vi "winchcontrol2014_preT-Tide_Altimeter_withTime.vi"() -> ()   [LabVIEW 2014]
uses:
  Instance           1 20Saved   winchcontrol .vi
  Instance           2 20Saved   winchcontrol .vi
  Instance           4 20Saved   winchcontrol .vi
  Instance           3 20Saved   winchcontrol .vi
  Instance           5 20Saved   winchcontrol .vi
  Instance           6 20Saved   winchcontrol .vi
panel:
  in  "pressure num":dbl
  out "Dz/Dt":T1(graph)
  in  "VelOut Fact.[turns/s]":dbl=4.2 min=0.0 max=8.0 step=0.1 format="%_2f"
  out "Depth History":T2(graph)
  out "Conductivity":T1(graph)
  out "Alti Range":T1(graph)
  in  "Path of Image Capture":path=path "/OPG_Winch_MiniCoreDuo/Users/opg/Sites/FCTD_WINCH/LabView.png"
  in  "Screen Capture":bool
  out "Last update string":string="Updated: 10/29/12 6:37:41 PM"
  in  "Port":i32=4050
  in  "Red Lion IP Address":string="192.168.1.160"
  in  "Beep\non wait?":bool=TRUE
  in  "Drive by \nCTD Data":bool=TRUE
  out "isMaxPaySet":bool
  out "Old Max Payout":dbl=500.0
  in  "Max. depth [m]":dbl=330.0 min=0.0 max=2000.0 step=1.0 format="%#_4f"
  out "Time @ max":timestamp=timestamp(3434357554.995505 s since 1904-01-01) format="%<%H:%M:%S>T"
  out "Max payout":dbl=26.1 format="%#_6f"
  out "Max depth":dbl format="%#_6f"
  in  "Go Up Now":bool
  in  "Final In Speed\n[turns/sec]":dbl=0.7 min=0.0 max=4.0 step=0.1 format="%_2f"
  in  "Slow depth\n[turns]":dbl=7.0 min=0.0 max=1500.0 step=1.0
  out "Final in Speed":dbl=0.7 min=0.0 max=4.0 step=0.1 format="%3_2g"
  out "Slow Depth":dbl=7.0 min=0.0 max=4.0 step=0.1
  out "CTD Com Miss Count":dbl
  out "Winch Com Miss Count":dbl=1.0
  out "Sax Status":u8[](array[numeric])=[1, 1, 0, 0, 5, 0, 1, 1, 0, 0]
  out "Pressure":T1(graph)
  out "i value":i32
  out "concatenated string":string="$OPGST,1,2,1243"
  out "CTD data":string="2615984408,1.818078,23.842880,5.097004"
  out "Depth":dbl(slide)=1.8080824462346528 min=0.0 max=1200.0 scale format="%#_4f"
  out "*(type *) &x":i32=38
  out "timestamp":u32=2615984408
  out "Temperature":T1(graph)
  out "Parameter String":string="$reqparmx:0019;0000$OPGWPM,10,16,+   6,+ 500, 4.2, 2.0,10000,10000,20000,40000,60000,60000,    0.70,    7,;"
  out "Status String":string="$OPGWST,3,1,+   1.8, 266.9,   0,- 0.01,   0.00,   0,   26307,;"
  out "Sax Status Code":dbl=26307.0 format="%#_8f"
  out "Motor Current":dbl
  out "Motor Payout":dbl=266.9
  out "Sheave Payout":dbl
  out "ATM90 Payout":dbl=1.8
  in  "CTD Data  IP Address":string="192.168.1.158"
  in  "Port":i32=2342
  out "bytes written":i32=62
  out "RL Status Received":bool=TRUE
  out "Acc Out":dbl=10000.0
  out "Acc In":dbl=10000.0
  out "Winch Action Status":T3(ring)=enum."HOMING"
  out "Winch Control Mode":u16(ring)=3 items=["STOPPED", "MANUAL JOY", "MANUAL POT", "AUTO", "SEMIAUTO"]
  out "Decel Stop In":dbl=60000.0
  out "Decel Stop Out":dbl=60000.0
  out "Decel In":dbl=40000.0
  out "Decel Out":dbl=20000.0
  out "Wire In Speed":dbl=2.0
  out "Wire Out Speed":dbl=4.2
  out "Min Payout":dbl=6.0
  out "Max Payout":dbl=500.0
  out "I Limit Out":dbl=10.0
  out "I Limit In":dbl=16.0
  in  "Drop time [min.]":dbl=8.099999999999985 min=0.0 step=0.1 format="%.1f"
  out "output":string
  in  "Stop Now":bool
  in  "Wire In Speed\n[turns/sec]":dbl=2.0 min=0.0 max=5.0 step=0.1 format="%3_2f"
  in  "Decel in":dbl=40000.0
  in  "Decel out":dbl=20000.0
  in  "Stop decel in":dbl=60000.0
  in  "Stop decel out":dbl=60000.0
  in  "Accel  in":dbl=10000.0
  in  "Accel out":dbl=10000.0
  in  "Current limit out\n[Amps]":dbl=10.0 min=0.0 max=20.0 step=0.1 format="%_3f"
  in  "Current limit in\n[Amps]":dbl=16.0 min=0.0 max=18.0 format="%_3f"
  out "input 2":string="$reqparmx:0019;0000$OPGWPM,10,16,+   6,+ 500, 4.2, 2.0,10000,10000,20000,40000,60000,60000,    0.70,    7,;"
  out "Payout":dbl(slide)=1.8 min=0.0 max=1200.0 step=200.0 scale format="%#1_3f"
  out "Velocity Now":dbl(knob)=-0.01 min=-5.0 max=5.0 step=1.0 scale=-5.0..5.0 scale format="%#_1f"
  in  "Max. payout [turns]":dbl=500.0 min=0.0 max=1640.0 step=1.0 format="%#_4f"
  in  "Min. payout [turns]":dbl=6.0 min=0.0 max=2000.0 step=1.0
  in  "Winch Auto Run":bool=TRUE
  out "Enabled":bool=TRUE
  in  "Wire Out Speed\n[turns/sec]":dbl=4.2 min=0.0 max=8.0 step=0.1 format="%_2f"
  out "Target\nDepth":dbl
  # "OPG  FAST  CTD"
  # "Winch Variable Status"
  # "Winch Variable Controls"
  # "FCTD DATA COMMUNICATION SETUP"
  # "RED LION CONTROL PANEL COM."
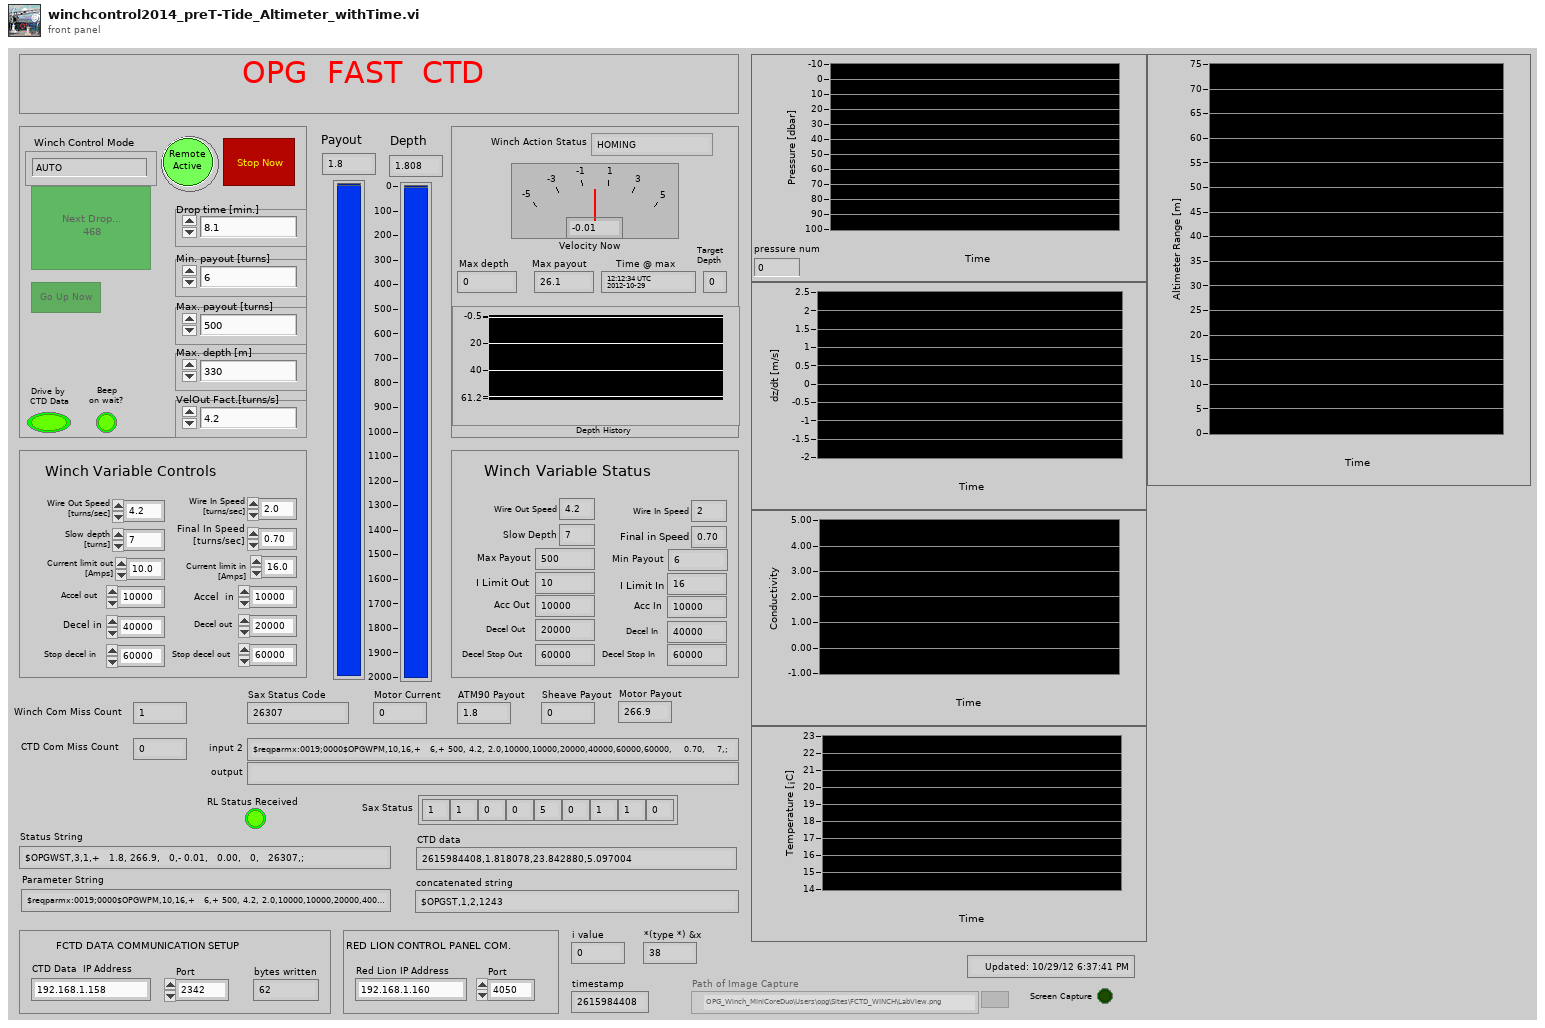
[diagram p1: front panel]
types:
  T1 = cluster{"seconds since 1Jan1904":timestamp, dbl}[]
  T2 = cluster{cluster{"seconds since 1Jan1904":dbl, dbl}[]}[]
  T3 = enum16{"START HOMING", "HOMING", "WAIT FOR TRIGGER", "START DROP", "GOING DOWN ?", "GOING UP"}
  T4 = cluster{"Array[0]":dbl, "Array[1]":dbl, "Array[2]":dbl, "Array[3]":dbl, "Array[4]":dbl, "Array[5]":dbl, "Array[6]":dbl, "Array[7]":dbl, "Array[8]":dbl}
  T5 = cluster{"Array[0]":dbl, "Array[1]":dbl, "Array[2]":dbl, "Array[3]":dbl, "Array[4]":dbl, "Array[5]":dbl, "Array[6]":dbl, "Array[7]":dbl, "Array[8]":dbl, "Array[9]":dbl, "Array[10]":dbl, "Array[11]":dbl, "Array[12]":dbl, "Array[13]":dbl}
  T6 = typedef "imagedata.ctl" = cluster{"image type":i32, "image depth":i32, "image":u8[], "mask":u8[], "colors":u32[], "Rectangle":cluster{"left":i16, "top":i16, "right":i16, "bottom":i16}}
  T7 = cluster{cluster{"seconds since 1Jan1904":dbl, dbl}[]}
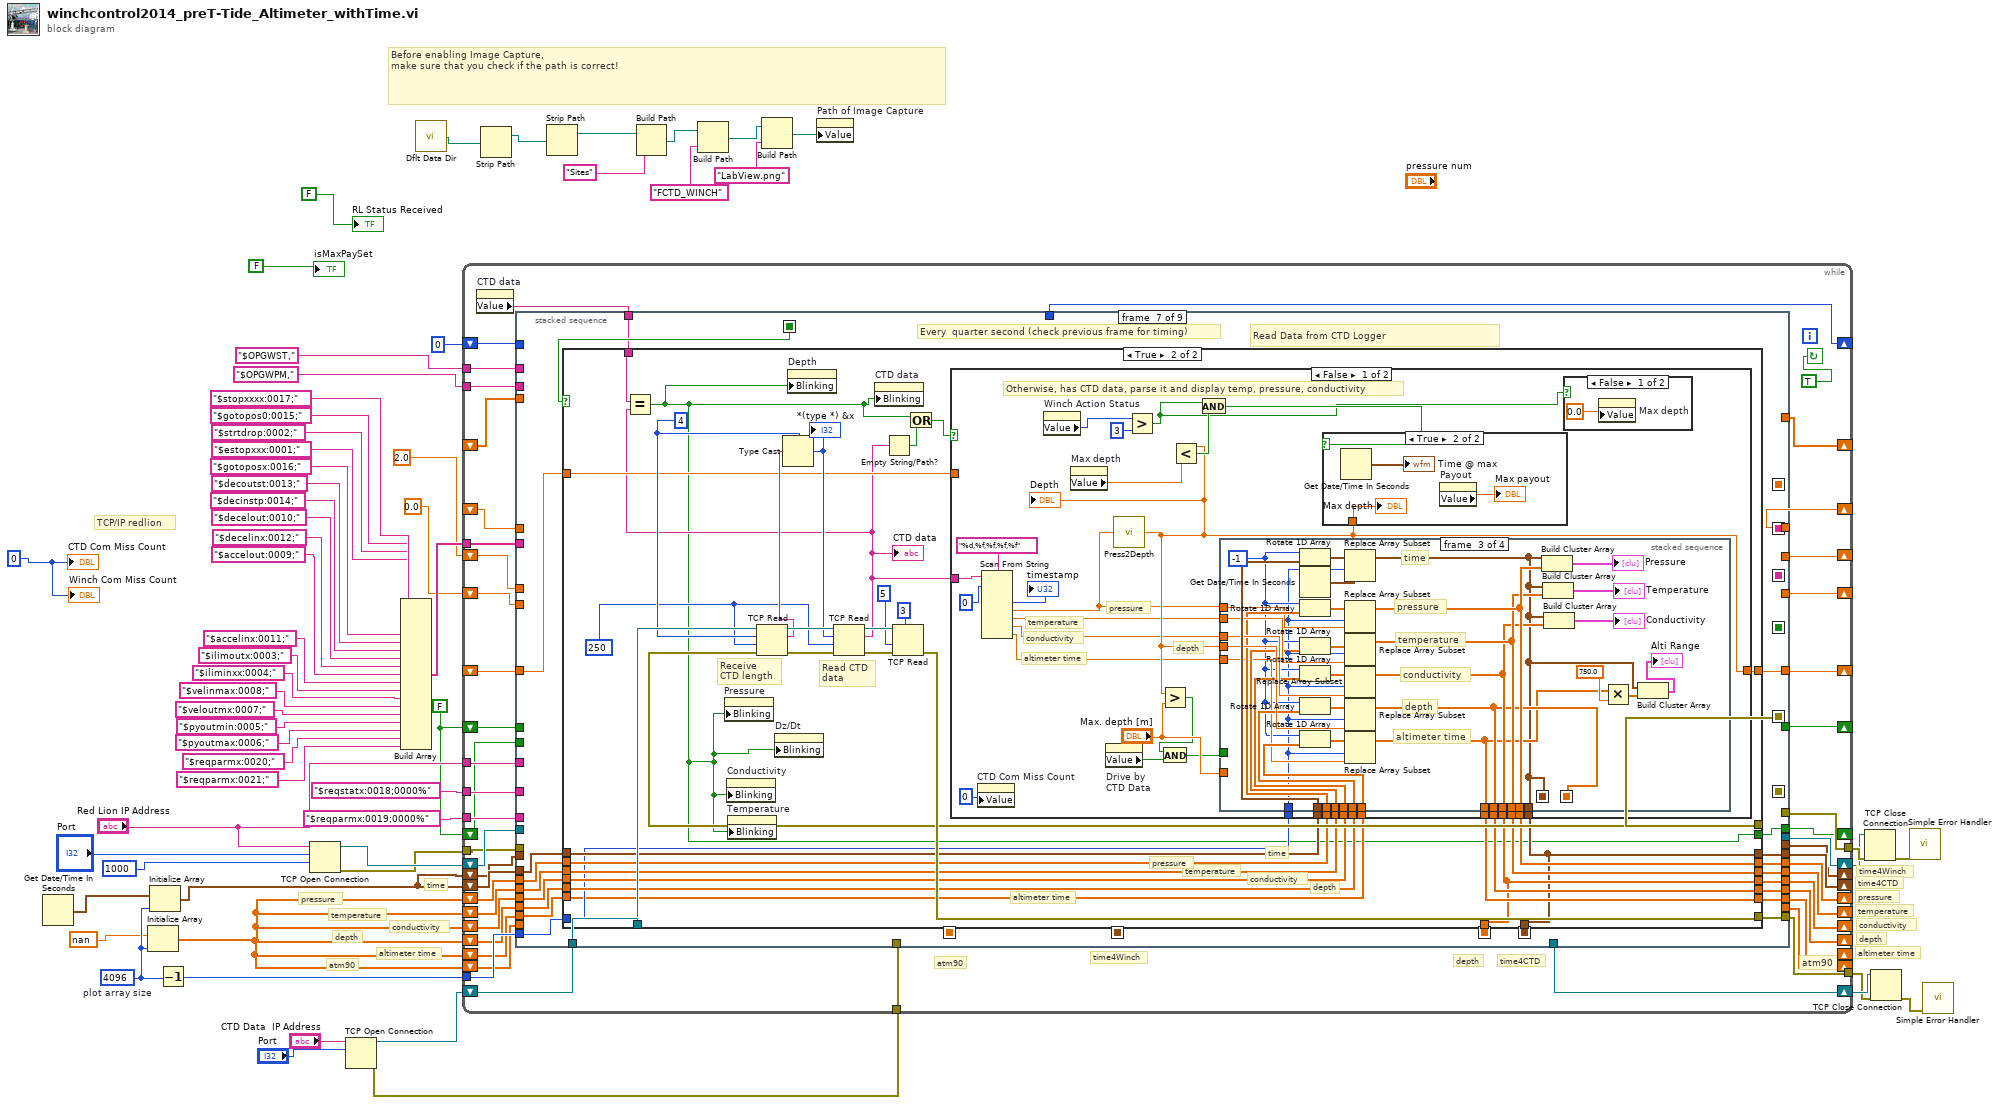
[diagram p0: block diagram]
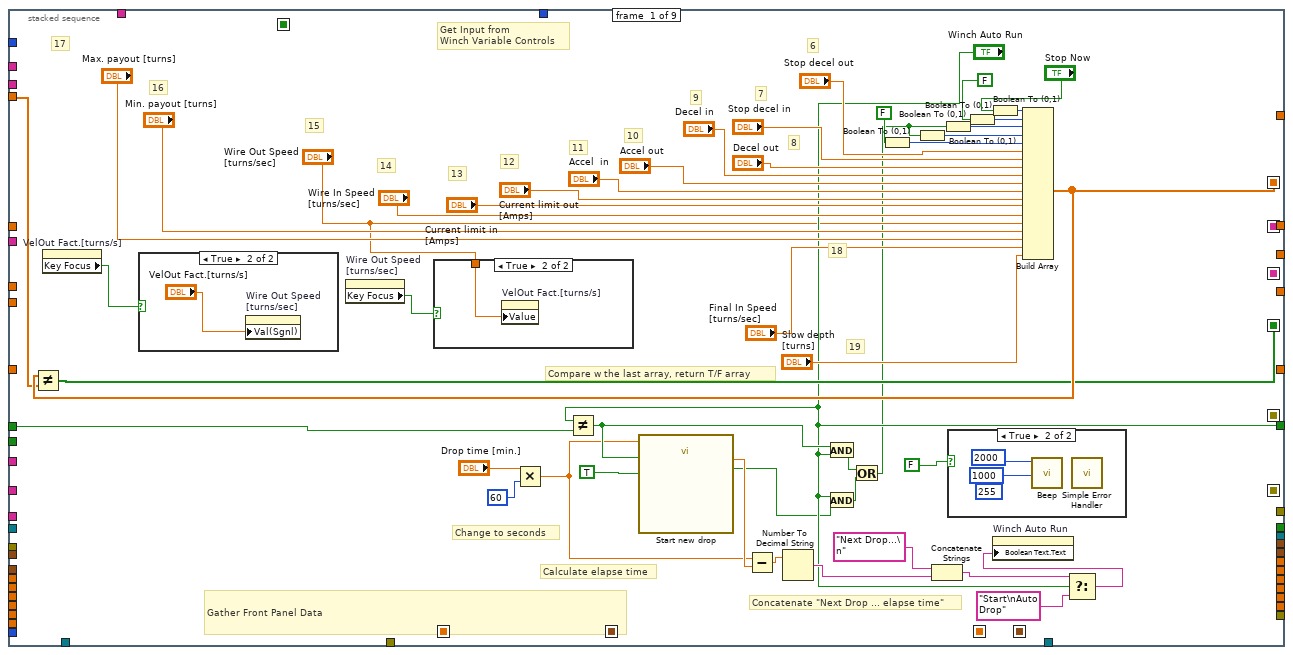
[diagram p2: hidden frame]
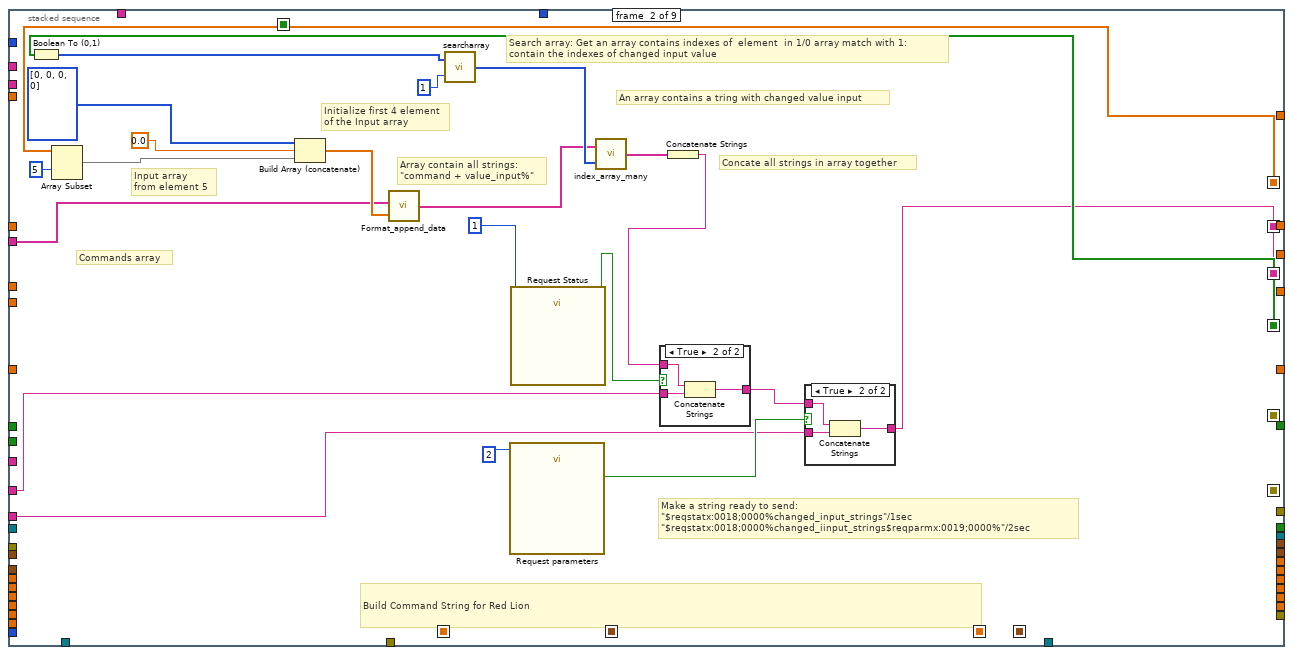
[diagram p6: hidden frame]
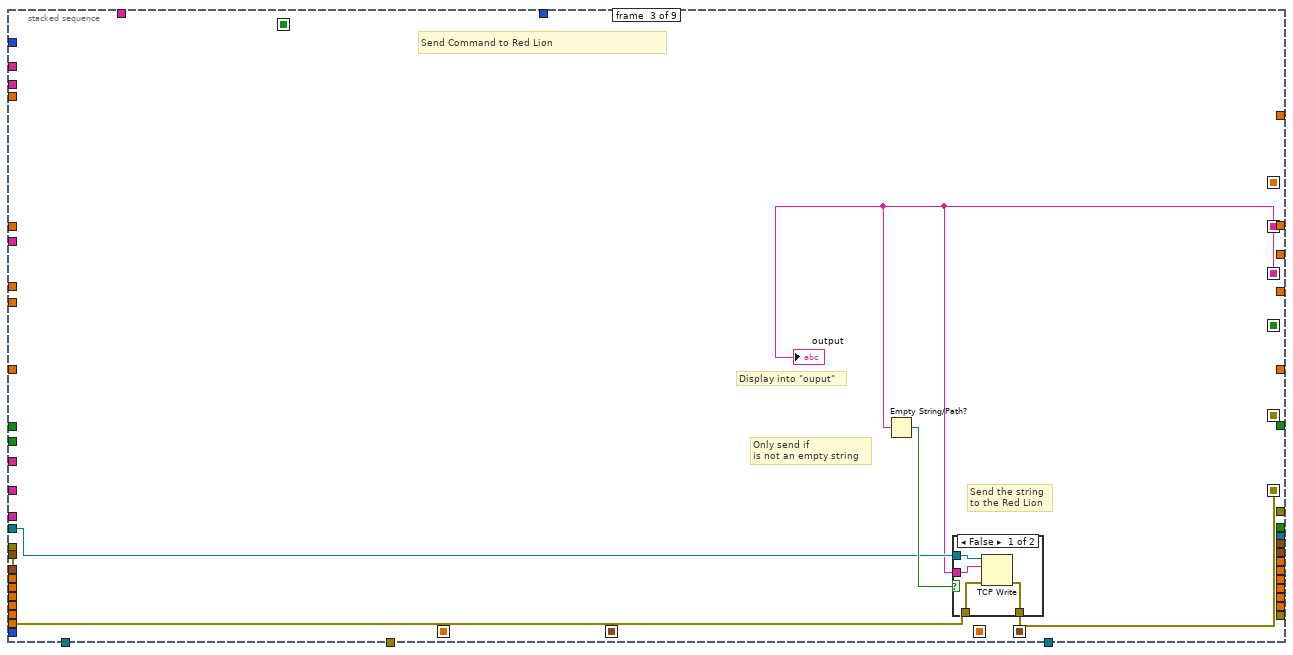
[diagram p9: hidden frame]
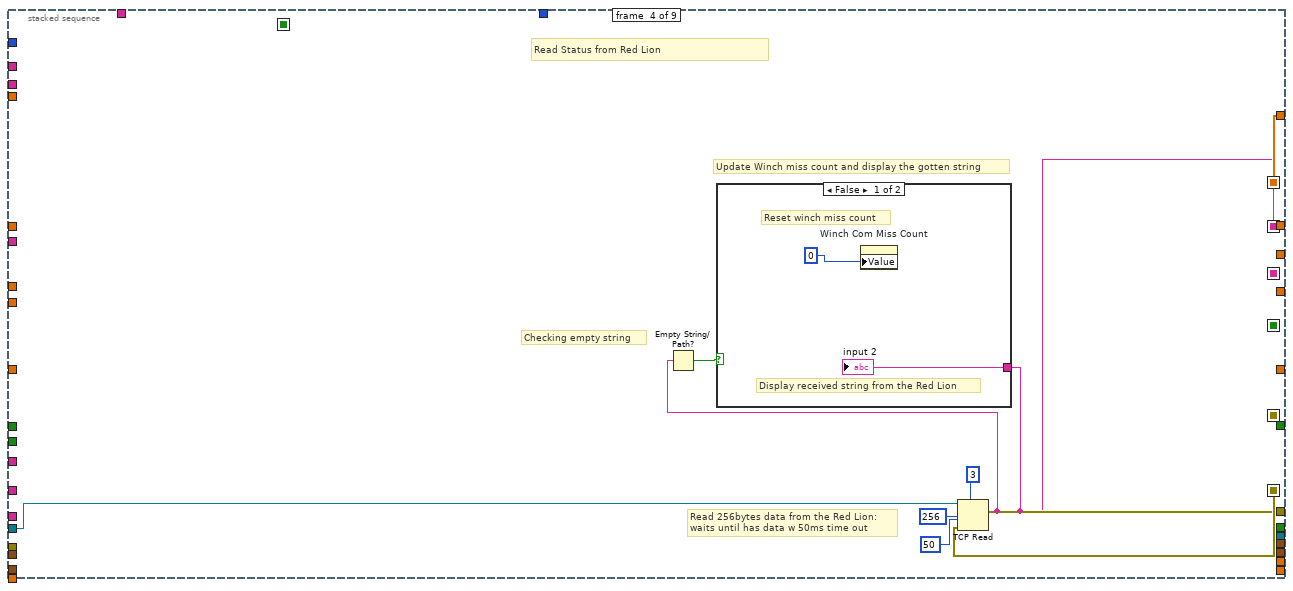
[diagram p11: hidden frame]
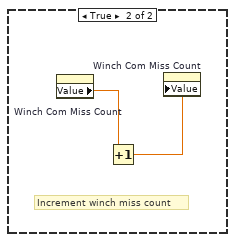
[diagram p12: hidden frame]
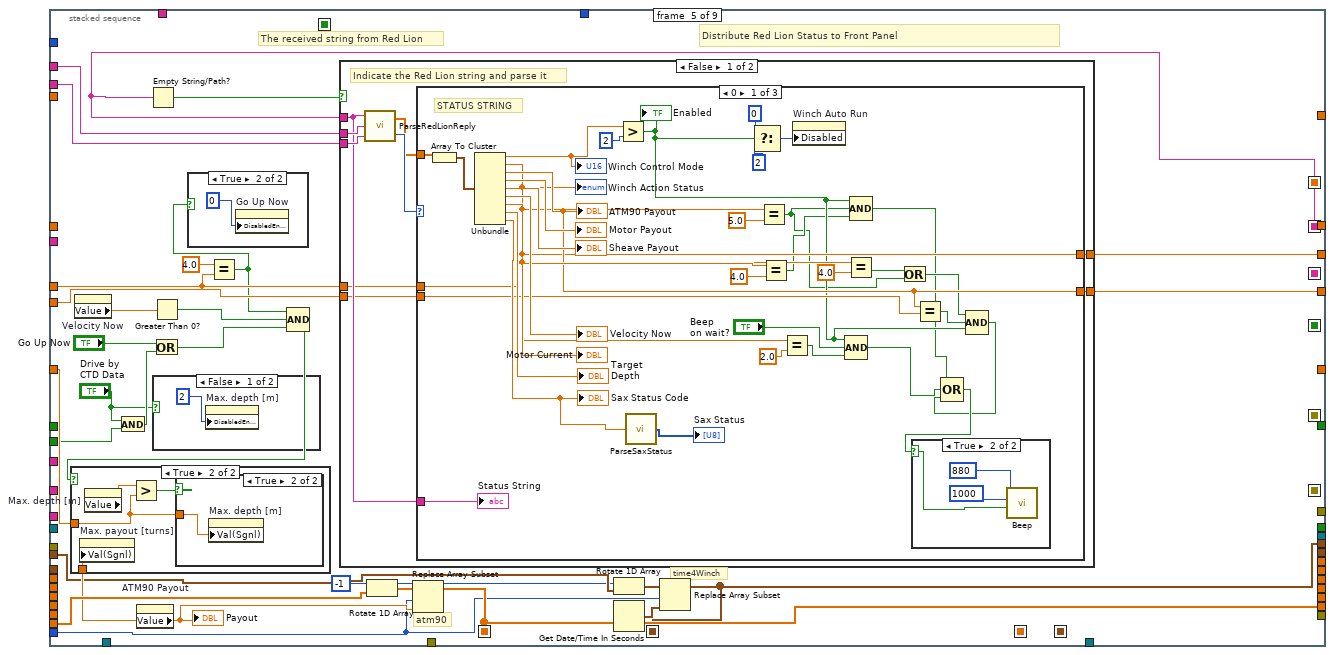
[diagram p13: hidden frame]
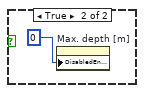
[diagram p14: hidden frame]
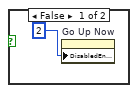
[diagram p15: hidden frame]
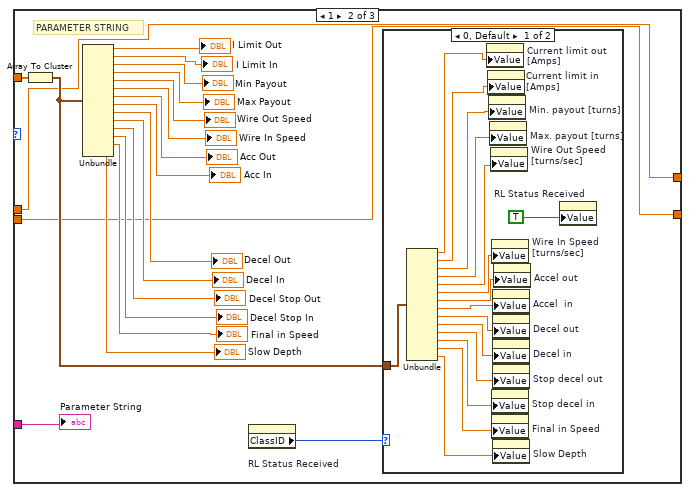
[diagram p19: hidden frame]
diagram:
  w5 = 4096  # plot array size
  w18 = FALSE
  w25 = 0
  # "time4Winch"
  # "atm90"
  # "depth"
  # "altimeter time"
  # "altimeter time"
  # "conductivity"
  # "temperature"
  # "time4CTD"
  # "pressure"
  # "depth"
  # "conductivity"
  # "temperature"
  # "time"
  # "pressure"
  # "Before enabling Image Capture, \nmake sure that you check if the path is correct!"
  # "TCP/IP redlion"
  n1 = Get Date/Time In Seconds() -> (seconds since 1Jan1904=w4:timestamp)
  n2 = Initialize Array(nan, w5) -> (w3:dbl[])
  n3 = Initialize Array(w4, w5) -> (w2:timestamp[])
  n4 = Decrement(x=w5) -> (x-1=w6:i32)
  n5 = TCP Open Connection(address="Red Lion IP Address", remote port or service name="Port", timeout ms (60000)=1000) -> (connection ID=w60:refnum<k5>, error out=w58:errorcluster)  [unwired: 2 in]
  n6 = TCP Open Connection(address="CTD Data  IP Address", remote port or service name="Port") -> (connection ID=w34:refnum<k5>, error out=w32:errorcluster)  [unwired: 3 in]
  n7 = Build Array("$stopxxxx:0017;", "$gotopos0:0015;", "$strtdrop:0002;", "$estopxxx:0001;", "$gotoposx:0016;", "$decoutst:0013;", "$decinstp:0014;", "$decelout:0010;", "$decelinx:0012;", "$accelout:0009;", "$accelinx:0011;", "$ilimoutx:0003;", "$iliminxx:0004;", "$velinmax:0008;", "$veloutmx:0007;", "$pyoutmin:0005;", "$pyoutmax:0006;", "$reqparmx:0020;", "$reqparmx:0021;") -> (w56:string[])
  n8 = call <vilib>:"Dflt Data Dir.vi"() -> ("App:Default Data Directory"=w15:path)
  n9 = while {
    shift-right: [w110] -> _
    shift-left: _ -> [w108]
    tunnel: w58 -> [w105]
    tunnel: [w109] -> w57
    tunnel: w56 -> [w107]
    tunnel: "$reqstatx:0018;0000%" -> [w104]
    shift-right: [w103] -> _
    shift-left: w18 -> [w102]
    tunnel: w32 -> [w100]
    tunnel: [w99] -> w31
    tunnel: "$reqparmx:0019;0000%" -> [w98]
    shift-right: [w97] -> _
    shift-left: _ -> [w96]
    shift-right: [w95] -> _
    shift-left: 0 -> [w94]
    tunnel: "$OPGWST," -> [w93]
    tunnel: "$OPGWPM," -> [w92]
    shift-right: [w90] -> w24
    shift-left: w60 -> [w106]
    shift-right: [w89] -> w33
    shift-left: w34 -> [w101]
    shift-right: [w88] -> _
    shift-left: _ -> [w87]
    tunnel: "Red Lion IP Address" -> [w85]
    shift-right: [w84] -> _
    shift-left: w18 -> [w83]
    shift-right: [w82] -> _
    shift-left: 2.0 -> [w81]
    shift-right: [w80] -> _
    shift-left: 0.0 -> [w79]
    tunnel: w6 -> [w78]
    shift-right: [w70] -> _
    shift-left: w3 -> [w76]
    shift-right: [w72] -> _
    shift-left: w2 -> [w77]
    shift-right: [w69] -> _
    shift-left: w3 -> [w75]
    shift-right: [w67] -> _
    shift-left: w3 -> [w74]
    shift-right: [w68] -> _
    shift-left: w3 -> [w73]
    shift-right: [w66] -> _
    shift-left: w3 -> [w71]
    shift-right: [w64] -> _
    shift-left: w3 -> [w65]
    shift-right: [w62] -> _
    shift-left: w2 -> [w63]
    stop <- TRUE continue-if-true
    # "time4CTD"
    # "time4Winch"
    # "depth"
    # "atm90"
    # "atm90"
    n10 = property on="CTD data" class="Str"() -> ("Value"=w86:string)  [unwired: 2 in, 2 out]
    n11 = stacked-sequence {
      seq-local: [w156 _ _ _ _ _ _ _ _] -> [_ w175 _ w209 _ _ _ _ _]
      seq-local: [_ w161 _ _ _ _ _ _ _] -> [_ _ w191 _ _ _ _ _ _]
      seq-local: [_ _ w192 _ _ _ _ _ _] -> [_ _ _ w204 _ _ _ _ _]
      seq-local: [w152 _ _ _ _ _ _ _ _] -> [_ w182 _ _ _ _ _ _ _]
      seq-local: [_ _ _ w202 _ _ _ _ _] -> [_ _ _ _ w240 _ _ _ _]
      seq-local: [_ _ _ _ _ w345 _ _ _] -> [_ _ _ _ _ _ w405 _ _]
      seq-local: [_ _ _ _ _ w344 _ _ _] -> [_ _ _ _ _ _ w403 _ _]
      seq-local: [_ _ _ _ _ _ w385 _ _] -> [_ _ _ _ _ _ _ _ w616]
      seq-local: [_ _ _ _ w219 _ _ _ _] -> [_ _ _ _ _ _ _ _ w617]
      seq-local: [_ _ _ _ w214 _ _ _ _] -> [_ _ _ _ _ _ _ _ w621]
      seq-local: [_ _ _ _ _ _ w384 _ _] -> [_ _ _ _ _ _ _ _ w620]
      tunnel: w105 -> [_ _ w194 _ _ _ _ _ _]
      tunnel: w106 -> [_ _ w193 w205 _ _ _ w581 _]
      tunnel: [_ _ _ w209 _ _ _ _ _] -> w110
      tunnel: w107 -> [_ w173 _ _ _ _ _ _ _]
      tunnel: [_ _ _ w203 _ _ _ _ _] -> w109
      tunnel: w108 -> [w155 _ _ _ _ _ _ _ _]
      tunnel: w104 -> [_ w167 _ _ _ _ _ _ _]
      tunnel: ["Winch Auto Run" _ _ _ _ _ _ _ _] -> w103
      tunnel: w102 -> [w131 _ _ _ _ _ _ _ _]
      tunnel: w101 -> [_ _ _ _ _ w347 w406 w579 _]
      tunnel: w100 -> [_ _ _ _ _ w346 _ _ _]
      tunnel: [_ _ _ _ _ _ w404 _ _] -> w99
      tunnel: w98 -> [_ w162 _ _ _ _ _ _ _]
      tunnel: [_ _ _ _ _ w343 _ _ _] -> w97
      tunnel: w96 -> [_ _ _ _ _ w342 _ _ _]
      tunnel: w94 -> [_ _ _ _ _ w341 _ _ _]
      tunnel: [_ _ _ _ _ w340 _ _ _] -> w95
      tunnel: w93 -> [_ _ _ _ w242 _ _ _ _]
      tunnel: w92 -> [_ _ _ _ w241 _ _ _ _]
      tunnel: [_ _ _ _ _ _ _ w580 _] -> w90
      tunnel: [_ _ _ _ _ _ _ w578 _] -> w89
      tunnel: [_ _ _ _ _ _ w402 _ _] -> w88
      tunnel: w87 -> [_ _ _ _ w235 _ w401 _ _]
      tunnel: w86 -> [_ _ _ _ _ _ w400 _ _]
      tunnel: w85 -> [_ _ _ _ _ _ _ w577 _]
      tunnel: [_ _ _ _ _ _ w399 _ _] -> w84
      tunnel: w83 -> [_ _ _ _ w232 _ _ _ _]
      tunnel: [_ _ _ _ w229 _ _ _ _] -> w82
      tunnel: w81 -> [_ _ _ _ w225 _ _ _ _]
      tunnel: [_ _ _ _ w228 _ _ _ _] -> w80
      tunnel: w79 -> [_ _ _ _ w227 _ _ _ _]
      tunnel: w78 -> [_ _ _ _ w216 _ w398 _ _]
      tunnel: w77 -> [_ _ _ _ _ _ w397 _ _]
      tunnel: w76 -> [_ _ _ _ _ _ w396 _ _]
      tunnel: w75 -> [_ _ _ _ _ _ w395 _ _]
      tunnel: w74 -> [_ _ _ _ _ _ w394 _ _]
      tunnel: w73 -> [_ _ _ _ _ _ w393 _ _]
      tunnel: [_ _ _ _ _ _ w392 _ _] -> w72
      tunnel: w71 -> [_ _ _ _ _ _ w391 _ _]
      tunnel: [_ _ _ _ _ _ w390 _ _] -> w70
      tunnel: [_ _ _ _ _ _ w389 _ _] -> w69
      tunnel: [_ _ _ _ _ _ w388 _ _] -> w67
      tunnel: [_ _ _ _ _ _ w387 _ _] -> w68
      tunnel: [_ _ _ _ _ _ w386 _ _] -> w66
      tunnel: w65 -> [_ _ _ _ w223 _ _ _ _]
      tunnel: [_ _ _ _ w219 _ _ _ _] -> w64
      tunnel: w63 -> [_ _ _ _ w218 _ _ _ _]
      tunnel: [_ _ _ _ w214 _ _ _ _] -> w62
      frame #0 {
        w153 = FALSE items=["OFF", "ON", "OFF", "ON"] ("Return to top")
        w140 = FALSE items=["OFF", "ON", "OFF", "ON"] ("Go to ...")
        # "19"
        # "18"
        # "17"
        # "16"
        # "15"
        # "14"
        # "13"
        # "12"
        # "11"
        # "10"
        # "9"
        # "8"
        # "7"
        # "6"
        # "Compare w the last array, return T/F array"
        # "Concatenate \"Next Drop ... elapse time\""
        # "Calculate elapse time"
        # "Change to seconds"
        # "Get Input from\nWinch Variable Controls"
        # "Gather Front Panel Data"
        n12 = property on="VelOut Fact.[turns/s]" class="DigNum (strict)"() -> ("Key Focus"=w114:bool)  [unwired: 2 in, 2 out]
        n13 = case shown="True" w114 {
          frame False {
          }
          frame True {
            n14 = property on="Wire Out Speed\n[turns/sec]" class="DigNum (strict)"("Val(Sgnl)"="VelOut Fact.[turns/s]") -> ()  [unwired: 2 in, 2 out]
          }
        }
        n15 = property on="Wire Out Speed\n[turns/sec]" class="DigNum (strict)"() -> ("Key Focus"=w113:bool)  [unwired: 2 in, 2 out]
        n16 = case shown="True" w113 {
          tunnel: "Wire Out Speed\n[turns/sec]" -> [_ w157]
          frame False {
          }
          frame True {
            n17 = property on="VelOut Fact.[turns/s]" class="DigNum (strict)"("Value"=w157) -> ()  [unwired: 2 in, 2 out]
          }
        }
        n18 = Multiply(x="Drop time [min.]", y=60) -> (x*y=w126:dbl)
        n19 = Not Equal?(x="Winch Auto Run", y=w131) -> (x != y?=w130:bool)
        n20 = call "Start new drop"("Time Target (s)"=w126, "Reset"=w130, "Auto Reset"=TRUE) -> ("Elapsed Time (s)"=w127:dbl, "Time has Elapsed"=w116:bool)  [unwired: 9 in, 6 out]
        n21 = Subtract(x=w126, y=w127) -> (x-y=w125:dbl)
        n22 = Number To Decimal String(number=w125) -> (decimal integer string=w124:string)  [unwired: 1 in]
        n23 = And(x=w130, y="Winch Auto Run") -> (x .and. y?=w129:bool)
        n24 = And(x="Winch Auto Run", y=w116) -> (x .and. y?=w128:bool)
        n25 = Or(x=w129, y=w128) -> (x .or. y?=w111:bool)
        n26 = Boolean To (0,1)(Boolean=w140) -> (0, 1=w139:i16)
        n27 = Boolean To (0,1)(Boolean=w111) -> (0, 1=w138:i16)
        n28 = Concatenate Strings("Next Drop...\n", w124) -> (w121:string)
        n29 = Boolean To (0,1)(Boolean=w111) -> (0, 1=w137:i16)
        n30 = case shown="True" FALSE {
          frame False {
          }
          frame True {
            (unwired) 255
            n31 = call <vilib>:"Beep.vi"("duration (msec) - ignored"=1000, "frequency (Hz) - ignored"=2000) -> ()  [unwired: 10 in]
            n32 = call <vilib>:"Simple Error Handler.vi"() -> ()  [unwired: 5 in, 5 out]
          }
        }
        n33 = Boolean To (0,1)(Boolean=w153) -> (0, 1=w136:i16)
        n34 = Boolean To (0,1)(Boolean="Stop Now") -> (0, 1=w135:i16)
        n35 = Build Array(w135, w136, w137, w138, w139, "Stop decel out", "Stop decel in", "Decel out", "Decel in", "Accel out", "Accel  in", "Current limit out\n[Amps]", "Current limit in\n[Amps]", "Wire In Speed\n[turns/sec]", "Wire Out Speed\n[turns/sec]", "Min. payout [turns]", "Max. payout [turns]", "Final In Speed\n[turns/sec]", "Slow depth\n[turns]") -> (w156:dbl[])
        n36 = Not Equal?(x=w156, y=w155) -> (x != y?=w152:bool[])
        n37 = Select(t=w121, s="Winch Auto Run", f="Start\nAuto Drop") -> (s? t:f=w122:string)
        n38 = property on="Winch Auto Run" class="Bool (strict)"("Boolean Text.Text"=w122) -> ()  [unwired: 2 in, 2 out]
      }
      frame #1 {
        # "Make a string ready to send:\n\"$reqstatx:0018;0000%changed_input_strings\"/1sec\n\"$reqstatx:0018;0000%changed_iinput_strings$reqparmx:0019;0000%\"/2sec"
        # "Concate all strings in array together"
        # "An array contains a tring with changed value input"
        # "Array contain all strings:\n\"command + value_input%\""
        # "Commands array"
        # "Initialize first 4 element\nof the Input array"
        # "Input array\nfrom element 5"
        # "Search array: Get an array contains indexes of  element  in 1/0 array match with 1:\ncontain the indexes of changed input value"
        # "Build Command String for Red Lion"
        n39 = Boolean To (0,1)(Boolean=w182) -> (0, 1=w180:i16[])
        n40 = Array Subset(array=w175, index=5) -> (w171:dbl[])  [unwired: 1 in]
        n41 = Build Array (concatenate)(i32[] [0, 0, 0, 0], 0.0 ("Depth to go to"), w171) -> (w174:dbl[])
        n42 = call "Format_append_data.vi"("Numbers to append"=w174, "Strings without numbers"=w173) -> ("Final Strings"=w172:string[])
        n43 = call "searcharray.vi"("Search character"=1, "Array 2"=w180) -> ("Array"=w179:i16[])
        n44 = call "Request parameters"("Time Target (s)"=2) -> ("Time has Elapsed"=w163:bool)  [unwired: 11 in, 7 out]
        n45 = call "Request Status"("Time Target (s)"=1) -> ("Time has Elapsed"=w168:bool)  [unwired: 11 in, 7 out]
        n46 = call "index_array_many.vi"("Lines of Array to grab"=w179, "String Array Input"=w172) -> ("Output array"=w178:string[])
        n47 = Concatenate Strings(w178) -> (w166:string)
        n48 = case shown="True" w168 {
          tunnel: w166 -> [w187 w190]
          tunnel: [w187 w189] -> w164
          tunnel: w167 -> [_ w188]
          frame False {
          }
          frame True {
            n49 = Concatenate Strings(w190, w188) -> (w189:string)
          }
        }
        n50 = case shown="True" w163 {
          tunnel: w164 -> [w183 w186]
          tunnel: [w183 w185] -> w161
          tunnel: w162 -> [_ w184]
          frame False {
          }
          frame True {
            n51 = Concatenate Strings(w186, w184) -> (w185:string)
          }
        }
      }
      frame #2 {
        # "Send the string\nto the Red Lion"
        # "Only send if\nis not an empty string"
        # "Display into \"ouput\""
        # "Send Command to Red Lion"
        n52 = Empty String/Path?(string/path=w191) -> (empty?=w195:bool)
        n53 = case shown="False" w195 {
          tunnel: w191 -> [w198 _]
          tunnel: w193 -> [w199 _]
          tunnel: w194 -> [w197 w200]
          tunnel: [w196 w200] -> w192
          frame False {
            n54 = TCP Write(connection ID=w199, data in=w198, error in (no error)=w197) -> (error out=w196:errorcluster)  [unwired: 1 in, 2 out]
          }
          frame True {
          }
        }
        "output" <- w191
      }
      frame #3 {
        # "Update Winch miss count and display the gotten string"
        # "Checking empty string"
        # "Read 256bytes data from the Red Lion:\nwaits until has data w 50ms time out"
        # "Read Status from Red Lion"
        n55 = TCP Read(connection ID=w205, bytes to read=256, error in (no error)=w204, 7:3, 9:50) -> (data out=w202:string, error out=w203:errorcluster)  [unwired: 1 out]
        n56 = Empty String/Path?(string/path=w202) -> (empty?=w201:bool)
        n57 = case shown="False" w201 {
          tunnel: w202 -> [w211 _]
          frame False {
            # "Display received string from the Red Lion"
            # "Reset winch miss count"
            n58 = property on="Winch Com Miss Count" class="DigNum (strict)"("Value"=0) -> ()  [unwired: 2 in, 2 out]
            "input 2" <- w211
          }
          frame True {
            # "Increment winch miss count"
            n59 = property on="Winch Com Miss Count" class="DigNum (strict)"() -> ("Value"=w213:dbl)  [unwired: 2 in, 2 out]
            n60 = Increment(x=w213) -> (x+1=w212:dbl)
            n61 = property on="Winch Com Miss Count" class="DigNum (strict)"("Value"=w212) -> ()  [unwired: 2 in, 2 out]
          }
        }
      }
      frame #4 {
        w217 = -1
        # "time4Winch"
        # "atm90"
        # "The received string from Red Lion"
        # "Distribute Red Lion Status to Front Panel"
        n62 = property on="Velocity Now" class="Knob (strict)"() -> ("Value"=w238:dbl)  [unwired: 2 in, 2 out]
        n63 = And(x="Drive by \nCTD Data", y=w232) -> (x .and. y?=w231:bool)
        n64 = property on="ATM90 Payout" class="DigNum (strict)"() -> ("Value"=w221:dbl)  [unwired: 2 in, 2 out]
        "Payout" <- w221
        n65 = Empty String/Path?(string/path=w240) -> (empty?=w239:bool)
        n66 = Greater Than 0?(x=w238) -> (x > 0?=w236:bool)
        n67 = Or(x="Go Up Now", y=w231) -> (x .or. y?=w233:bool)
        n68 = case shown="False" "Drive by \nCTD Data" {
          frame False {
            n69 = property on="Max. depth [m]" class="DigNum (strict)"("DisabledEnum"=2) -> ()  [unwired: 2 in, 2 out]
          }
          frame True {
            n70 = property on="Max. depth [m]" class="DigNum (strict)"("DisabledEnum"=0) -> ()  [unwired: 2 in, 2 out]
          }
        }
        n71 = Equal?(x=4.0, y=w225) -> (x = y?=w224:bool)
        n72 = case shown="True" w224 {
          frame False {
            n73 = property on="Go Up Now" class="Bool"("DisabledEnum"=2) -> ()  [unwired: 2 in, 2 out]
          }
          frame True {
            n74 = property on="Go Up Now" class="Bool"("DisabledEnum"=0) -> ()  [unwired: 2 in, 2 out]
          }
        }
        n75 = Compound Arithmetic op=AND(w224, w236, w233) -> (w237:bool)
        n76 = case shown="True" w237 {
          tunnel: w221 -> [_ w250]
          tunnel: w235 -> [_ w247]
          frame False {
          }
          frame True {
            n77 = property on="Max. payout [turns]" class="DigNum (strict)"("Val(Sgnl)"=w250) -> ()  [unwired: 2 in, 2 out]
            n78 = property on="Max. depth [m]" class="DigNum (strict)"() -> ("Value"=w249:dbl)  [unwired: 2 in, 2 out]
            n79 = Greater?(x=w249, y=w247) -> (0:w248:bool)
            n80 = case shown="True" w248 {
              tunnel: w247 -> [_ w251]
              frame False {
              }
              frame True {
                n81 = property on="Max. depth [m]" class="DigNum (strict)"("Val(Sgnl)"=w251) -> ()  [unwired: 2 in, 2 out]
              }
            }
          }
        }
        n82 = case shown="False" w239 {
          tunnel: w242 -> [w258 _]
          tunnel: w241 -> [w257 _]
          tunnel: w240 -> [w256 _]
          tunnel: [w255 w338] -> w229
          tunnel: w225 -> [w254 w338]
          tunnel: [w253 w337] -> w228
          tunnel: w227 -> [w252 w337]
          frame False {
            # "Indicate the Red Lion string and parse it"
            n83 = call "ParseRedLionReply.vi"("Parameter Iidicator"=w257, "Status Indicator"=w258, "Red Lion String"=w256) -> ("Type"=w260:i16, "Array"=w259:dbl[])
            n84 = case shown="0" w260 {
              tunnel: w259 -> [w294 w318 _]
              tunnel: w256 -> [w286 w304 _]
              tunnel: [w273 w301 w336] -> w255
              tunnel: w254 -> [w277 w301 w336]
              tunnel: [w276 w300 w335] -> w253
              tunnel: w252 -> [w275 w300 w335]
              frame 0 {
                # "STATUS STRING"
                n85 = Array To Cluster(array=w294) -> (cluster=w293:T4)
                n86 = Unbundle(w293) -> ("Array[0]"=w292:dbl, "Array[1]"=w273:dbl, "Array[2]"=w276:dbl, "Array[3]"=→"Motor Payout":dbl, "Array[4]"=→"Sheave Payout":dbl, "Array[5]"=→"Velocity Now":dbl, "Array[6]"=→"Motor Current":dbl, "Array[7]"=→"Target\nDepth":dbl, "Array[8]"=w282:dbl)
                "Winch Control Mode" <- w292
                "Winch Action Status" <- w273
                "ATM90 Payout" <- w276
                "Sax Status Code" <- w282
                n87 = Greater?(x=w292, y=2) -> (0:w269:bool)
                "Enabled" <- w269
                n88 = call "ParseSaxStatus.vi"("Status Code In"=w282) -> ("Status Flags"=→"Sax Status":i8[])
                n89 = Select(t=0, s=w269, f=2) -> (s? t:f=w283:i32)
                n90 = Equal?(x=w273, y=5.0) -> (x = y?=w262:bool)
                n91 = Equal?(x=w277, y=4.0) -> (x = y?=w266:bool)
                n92 = Equal?(x=w273, y=2.0) -> (x = y?=w268:bool)
                n93 = property on="Winch Auto Run" class="Bool (strict)"("Disabled"=w283) -> ()  [unwired: 2 in, 2 out]
                n94 = Compound Arithmetic op=AND(w269, "Beep\non wait?", w268) -> (w263:bool)
                n95 = Equal?(x=w273, y=4.0) -> (x = y?=w272:bool)
                n96 = Compound Arithmetic op=AND(w269, w262, w266) -> (w265:bool)
                n97 = Or(x=w272, y=w262) -> (x .or. y?=w271:bool)
                n98 = Equal?(x=w276, y=w275) -> (x = y?=w270:bool)
                n99 = Compound Arithmetic op=AND(w271, w270, w269) -> (w261:bool)
                n100 = Compound Arithmetic op=OR(w265, w263, w261) -> (w264:bool)
                n101 = case shown="True" w264 {
                  selector: w264 -> [_ w296]
                  frame False {
                  }
                  frame True {
                    n102 = call <vilib>:"Beep.vi"("use system alert? (T) - ignored"=w296, "duration (msec) - ignored"=u32 1000, "frequency (Hz) - ignored"=u32 880) -> ()  [unwired: 9 in]
                  }
                }
                "Status String" <- w286
              }
              frame 1 {
                # "PARAMETER STRING"
                n103 = Array To Cluster(array=w318) -> (cluster=w305:T5)
                n104 = Unbundle(w305) -> ("Array[0]"=→"I Limit Out":dbl, "Array[1]"=→"I Limit In":dbl, "Array[2]"=→"Min Payout":dbl, "Array[3]"=→"Max Payout":dbl, "Array[4]"=→"Wire Out Speed":dbl, "Array[5]"=→"Wire In Speed":dbl, "Array[6]"=→"Acc Out":dbl, "Array[7]"=→"Acc In":dbl, "Array[8]"=→"Decel Out":dbl, "Array[9]"=→"Decel In":dbl, "Array[10]"=→"Decel Stop Out":dbl, "Array[11]"=→"Decel Stop In":dbl, "Array[12]"=→"Final in Speed":dbl, "Array[13]"=→"Slow Depth":dbl)
                n105 = property on="RL Status Received" class="Bool (strict)"() -> ("ClassID"=w299:u32)  [unwired: 2 in, 2 out]
                n106 = case shown="0, Default" w299 {
                  tunnel: w305 -> [w334 _]
                  frame 0, Default {
                    n107 = Unbundle(w334) -> ("Array[0]"=w333:dbl, "Array[1]"=w332:dbl, "Array[2]"=w331:dbl, "Array[3]"=w330:dbl, "Array[4]"=w329:dbl, "Array[5]"=w328:dbl, "Array[6]"=w322:dbl, "Array[7]"=w327:dbl, "Array[8]"=w326:dbl, "Array[9]"=w325:dbl, "Array[10]"=w324:dbl, "Array[11]"=w323:dbl, "Array[12]"=w321:dbl, "Array[13]"=w320:dbl)
                    n108 = property on="Current limit out\n[Amps]" class="DigNum (strict)"("Value"=w333) -> ()  [unwired: 2 in, 2 out]
                    n109 = property on="Current limit in\n[Amps]" class="DigNum (strict)"("Value"=w332) -> ()  [unwired: 2 in, 2 out]
                    n110 = property on="Min. payout [turns]" class="DigNum (strict)"("Value"=w331) -> ()  [unwired: 2 in, 2 out]
                    n111 = property on="Max. payout [turns]" class="DigNum (strict)"("Value"=w330) -> ()  [unwired: 2 in, 2 out]
                    n112 = property on="Wire Out Speed\n[turns/sec]" class="DigNum (strict)"("Value"=w329) -> ()  [unwired: 2 in, 2 out]
                    n113 = property on="Wire In Speed\n[turns/sec]" class="DigNum (strict)"("Value"=w328) -> ()  [unwired: 2 in, 2 out]
                    n114 = property on="Stop decel in" class="DigNum (strict)"("Value"=w323) -> ()  [unwired: 2 in, 2 out]
                    n115 = property on="Final in Speed" class="DigNum (strict)"("Value"=w321) -> ()  [unwired: 2 in, 2 out]
                    n116 = property on="Accel  in" class="DigNum (strict)"("Value"=w327) -> ()  [unwired: 2 in, 2 out]
                    n117 = property on="Decel out" class="DigNum (strict)"("Value"=w326) -> ()  [unwired: 2 in, 2 out]
                    n118 = property on="Decel in" class="DigNum (strict)"("Value"=w325) -> ()  [unwired: 2 in, 2 out]
                    n119 = property on="Stop decel out" class="DigNum (strict)"("Value"=w324) -> ()  [unwired: 2 in, 2 out]
                    n120 = property on="Slow Depth" class="DigNum (strict)"("Value"=w320) -> ()  [unwired: 2 in, 2 out]
                    n121 = property on="Accel out" class="DigNum (strict)"("Value"=w322) -> ()  [unwired: 2 in, 2 out]
                    n122 = property on="RL Status Received" class="Bool (strict)"("Value"=TRUE) -> ()  [unwired: 2 in, 2 out]
                  }
                  frame 1 {
                  }
                }
                "Parameter String" <- w304
              }
              frame 2, Default {
                # "INVALID STRING"
              }
            }
          }
          frame True {
            # "If empty string, do nothing"
          }
        }
        n123 = Rotate 1D Array(1:w223, 2:w217) -> (0:w222:dbl[])
        n124 = Replace Array Subset(array=w222, new element=w221, index=w216) -> (w219:dbl[])
        n125 = Rotate 1D Array(1:w218, 2:w217) -> (0:w220:timestamp[])
        n126 = Get Date/Time In Seconds() -> (seconds since 1Jan1904=w215:timestamp)
        n127 = Replace Array Subset(array=w220, new element=w215, index=w216) -> (w214:timestamp[])
      }
      frame #5 {
        # "Time between\n each\nrequest for \nCTD data"
        # "Send Status to CTD Logger"
        n128 = call "Send to FastCTD  logger"("Time Target (s)"=0.25) -> ("Time has Elapsed"=w344:bool)  [unwired: 11 in, 7 out]
        n129 = case shown="True" w344 {
          tunnel: w347 -> [_ w360]
          tunnel: w346 -> [w350 w359]
          tunnel: [w350 w358] -> w345
          tunnel: [w349 w354] -> w343
          tunnel: w342 -> [w349 w353]
          tunnel: w341 -> [w348 w352]
          tunnel: [w348 w351] -> w340
          frame False {
          }
          frame True {
            n130 = property on="Status String" class="Str"() -> ("Value"=w356:string)  [unwired: 2 in, 2 out]
            n131 = Empty String/Path?(string/path=w356) -> (empty?=w357:bool)
            n132 = case shown="True" w357 {
              tunnel: w356 -> [w364 _]
              tunnel: [w364 w374] -> w355
              tunnel: [w363 w368] -> w354
              tunnel: w353 -> [w363 w367]
              tunnel: w352 -> [w362 w366]
              tunnel: [w362 w365] -> w351
              frame False {
              }
              frame True {
                # "Since Status string is empty, make a string \"$OPGST,1,2/3,1243\"\nto send to FCTD app"
                n133 = Increment(x=w366) -> (x+1=w365:i32)
                n134 = Quotient & Remainder(x=w365, y=4) -> (x-y*floor(x/y)=w371:i32)  [unwired: 1 out]
                n135 = Equal To 0?(x=w371) -> (x = 0?=w370:bool)
                n136 = case shown="False" w370 {
                  tunnel: [w377 w379] -> w369
                  tunnel: [w377 w379] -> w368
                  tunnel: w367 -> [w377 w378]
                  frame False {
                  }
                  frame True {
                    n137 = Equal?(x=w378, y=3.0) -> (x = y?=w380:bool)
                    n138 = Select(t=2.0 ("y"), s=w380, f=3.0 ("y")) -> (s? t:f=w379:dbl)
                  }
                }
                n139 = Number To Decimal String(number=w369) -> (decimal integer string=w373:string)  [unwired: 1 in]
                n140 = Concatenate Strings("$OPGST,1," ("string"), w373, ",1243" ("string")) -> (w374:string)
                "concatenated string" <- w374
              }
            }
            n141 = TCP Write(connection ID=w360, data in=w355, error in (no error)=w359) -> (bytes written=→"bytes written":i32, error out=w358:errorcluster)  [unwired: 1 in, 1 out]
          }
        }
        "i value" <- w341
      }
      frame #6 {
        # "Every  quarter second (check previous frame for timing)"
        # "Read Data from CTD Logger"
        n142 = case shown="True" w403 {
          selector: w403 -> [w413 _]
          tunnel: w406 -> [_ w448]
          tunnel: w405 -> [w415 w433]
          tunnel: [w415 w441] -> w404
          tunnel: [w414 w437] -> w402
          tunnel: w401 -> [w414 w436]
          tunnel: w400 -> [_ w434]
          tunnel: [w413 w418] -> w399
          tunnel: w398 -> [_ w426]
          tunnel: w397 -> [w408 w431]
          tunnel: w396 -> [w412 w430]
          tunnel: w395 -> [w411 w429]
          tunnel: w394 -> [w410 w428]
          tunnel: w393 -> [w407 w427]
          tunnel: [w408 w419] -> w392
          tunnel: w391 -> [w409 w425]
          tunnel: [w412 w424] -> w390
          tunnel: [w411 w423] -> w389
          tunnel: [w410 w420] -> w388
          tunnel: [w407 w422] -> w387
          tunnel: [w409 w421] -> w386
          tunnel: [w407 w420] -> w385
          tunnel: [w408 w419] -> w384
          frame False {
          }
          frame True {
            w432 = 250
            w447 = 4
            # "altimeter time"
            # "depth"
            # "conductivity"
            # "temperature"
            # "time"
            # "pressure"
            # "Read CTD\ndata"
            # "Receive\nCTD length"
            n143 = TCP Read(connection ID=w448, bytes to read=w447, error in (no error)=w433, 9:w432) -> (connection ID out=w446:refnum<k5>, data out=w445:string, error out=w443:errorcluster)  [unwired: 1 in]
            n144 = Type Cast(type=w447, x=w445) -> (*(type *) &x=w444:i32)
            "*(type *) &x" <- w444
            n145 = TCP Read(connection ID=w446, bytes to read=w444, error in (no error)=w443, 9:w432) -> (connection ID out=w440:refnum<k5>, data out=w435:string, error out=w442:errorcluster)  [unwired: 1 in]
            "CTD data" <- w435
            n146 = Equal?(x=w434, y=w435) -> (x = y?=w418:bool)
            n147 = property on="Pressure" class="XYGraph (strict)"("Blinking"=w418) -> ()  [unwired: 2 in, 2 out]
            n148 = property on="Conductivity" class="XYGraph (strict)"("Blinking"=w418) -> ()  [unwired: 2 in, 2 out]
            n149 = property on="Temperature" class="XYGraph (strict)"("Blinking"=w418) -> ()  [unwired: 2 in, 2 out]
            n150 = property on="Dz/Dt" class="XYGraph (strict)"("Blinking"=w418) -> ()  [unwired: 2 in, 2 out]
            n151 = property on="Depth" class="Slide (strict)"("Blinking"=w418) -> ()  [unwired: 2 in, 2 out]
            n152 = property on="CTD data" class="Str"("Blinking"=w418) -> ()  [unwired: 2 in, 2 out]
            n153 = Empty String/Path?(string/path=w435) -> (empty?=w417:bool)
            n154 = TCP Read(connection ID=w440, error in (no error)=w442, 7:3, 9:5) -> (error out=w441:errorcluster)  [unwired: 1 in, 2 out]
            n155 = Or(x=w418, y=w417) -> (x .or. y?=w416:bool)
            n156 = case shown="False" w416 {
              tunnel: w435 -> [w478 _]
              tunnel: [w466 w575] -> w437
              tunnel: w436 -> [_ w575]
              tunnel: w431 -> [w465 w572]
              tunnel: w430 -> [w464 w571]
              tunnel: w429 -> [w463 w570]
              tunnel: w428 -> [w462 w569]
              tunnel: w427 -> [w461 w568]
              tunnel: w426 -> [w460 _]
              tunnel: [w459 w572] -> w419
              tunnel: w425 -> [w458 w567]
              tunnel: [w456 w571] -> w424
              tunnel: [w454 w570] -> w423
              tunnel: [w451 w569] -> w420
              tunnel: [w450 w568] -> w422
              tunnel: [w449 w567] -> w421
              frame False {
                # "depth"
                # "altimeter time"
                # "conductivity"
                # "temperature"
                # "pressure"
                # "Otherwise, has CTD data, parse it and display temp, pressure, conductivity"
                n157 = property on="CTD Com Miss Count" class="DigNum (strict)"("Value"=0) -> ()  [unwired: 2 in, 2 out]
                n158 = Scan From String(format string="%d,%f,%f,%f,%f", input string=w478, initial scan location=u32 0) -> (output 1=→"timestamp":u32, output 2=w457:dbl, output 3=w455:dbl, output 4=w453:dbl, output 5=w452:dbl)  [unwired: 6 in, 3 out]
                n159 = property on="Winch Action Status" class="Enum (strict)"() -> ("Value"=w473:T3)  [unwired: 2 in, 2 out]
                n160 = property on="Max depth" class="DigNum (strict)"() -> ("Value"=w471:dbl)  [unwired: 2 in, 2 out]
                n161 = property on="Drive by \nCTD Data" class="Bool (strict)"() -> ("Value"=w474:bool)  [unwired: 2 in, 2 out]
                n162 = call "Press2Depth.vi"("Pressure in dbars"=w457) -> ("Depth in meters"=w466:dbl)
                "Depth" <- w466
                n163 = Greater?(x=w473, y=3) -> (0:w468:bool)
                n164 = Greater?(x=w466, y="Max. depth [m]") -> (0:w475:bool)
                n165 = And(x=w475, y=w474) -> (x .and. y?=w476:bool)
                n166 = Less?(x=w471, y=w466) -> (x < y?=w470:bool)
                n167 = And(x=w468, y=w470) -> (x .and. y?=w469:bool)
                n168 = stacked-sequence {
                  seq-local: [_ _ w515 _] -> [_ _ _ w545]
                  seq-local: [_ _ w511 _] -> [_ _ _ w544]
                  tunnel: w466 -> [_ w501 w533 _]
                  tunnel: "Max. depth [m]" -> [_ w503 _ _]
                  tunnel: w476 -> [w483 _ _ _]
                  tunnel: w465 -> [_ _ w541 _]
                  tunnel: w464 -> [_ _ w530 _]
                  tunnel: w463 -> [_ _ w531 _]
                  tunnel: w462 -> [_ _ w532 _]
                  tunnel: w461 -> [_ _ w529 _]
                  tunnel: w460 -> [_ _ w516 _]
                  tunnel: [_ _ w511 _] -> w459
                  tunnel: w458 -> [_ _ w526 _]
                  tunnel: w457 -> [_ _ w528 _]
                  tunnel: [_ _ w522 _] -> w456
                  tunnel: w455 -> [_ _ w536 _]
                  tunnel: [_ _ w520 _] -> w454
                  tunnel: w453 -> [_ _ w534 _]
                  tunnel: w452 -> [_ _ w524 _]
                  tunnel: [_ _ w517 _] -> w451
                  tunnel: [_ _ w515 _] -> w450
                  tunnel: [_ _ w513 _] -> w449
                  frame #0 {
                    n169 = case shown="True" w483 {
                      frame False {
                      }
                      frame True {
                        n170 = property on="isMaxPaySet" class="Bool (strict)"() -> ("Value"=w489:bool)  [unwired: 2 in, 2 out]
                        n171 = Not(x=w489) -> (.not. x?=w488:bool)
                        n172 = property on="Payout" class="Slide (strict)"() -> ("Value"=w491:dbl)  [unwired: 2 in, 2 out]
                        n173 = property on="Max. payout [turns]" class="DigNum (strict)"() -> ("Value"=w490:dbl)  [unwired: 2 in, 2 out]
                        n174 = property on="Velocity Now" class="Knob (strict)"() -> ("Value"=w487:dbl)  [unwired: 2 in, 2 out]
                        n175 = Less?(x=w491, y=w490) -> (x < y?=w484:bool)
                        n176 = Greater Or Equal To 0?(x=w487) -> (x >= 0?=w485:bool)
                        n177 = And(x=w485, y=w484) -> (x .and. y?=w486:bool)
                        n178 = case shown="True" w488 {
                          selector: w488 -> [_ w492]
                          frame False {
                          }
                          frame True {
                            n179 = property on="isMaxPaySet" class="Bool (strict)"("Val(Sgnl)"=w492) -> ()  [unwired: 2 in, 2 out]
                            n180 = property on="Max. payout [turns]" class="DigNum (strict)"() -> ("Value"=→"Old Max Payout":dbl)  [unwired: 2 in, 2 out]
                          }
                        }
                        n181 = case shown="True" w486 {
                          tunnel: w491 -> [_ w495]
                          frame False {
                          }
                          frame True {
                            n182 = Multiply(x=w495, y=0.8) -> (x*y=w494:dbl)
                            n183 = property on="Max. payout [turns]" class="DigNum (strict)"("Val(Sgnl)"=w494) -> ()  [unwired: 2 in, 2 out]
                          }
                        }
                      }
                    }
                  }
                  frame #1 {
                    n184 = property on="Velocity Now" class="Knob (strict)"() -> ("Value"=w506:dbl)  [unwired: 2 in, 2 out]
                    n185 = property on="isMaxPaySet" class="Bool (strict)"() -> ("Value"=w499:bool)  [unwired: 2 in, 2 out]
                    n186 = Multiply(x=w503, y=0.8) -> (x*y=w502:dbl)
                    n187 = Greater?(x=w501, y=w502) -> (0:w500:bool)
                    n188 = Less Than 0?(x=w506) -> (x < 0?=w505:bool)
                    n189 = And(x=w505, y=w500) -> (x .and. y?=w498:bool)
                    n190 = And(x=w499, y=w498) -> (x .and. y?=w497:bool)
                    n191 = case shown="True" w497 {
                      selector: w497 -> [_ w508]
                      frame False {
                      }
                      frame True {
                        # "temporary store\nold payout to set\nsmall payout for\nfish to go up"
                        n192 = Not(x=w508) -> (.not. x?=w507:bool)
                        n193 = property on="isMaxPaySet" class="Bool (strict)"("Val(Sgnl)"=w507) -> ()  [unwired: 2 in, 2 out]
                        n194 = property on="Old Max Payout" class="DigNum (strict)"() -> ("Value"=w509:dbl)  [unwired: 2 in, 2 out]
                        n195 = property on="Max. payout [turns]" class="DigNum (strict)"("Val(Sgnl)"=w509) -> ()  [unwired: 2 in, 2 out]
                      }
                    }
                  }
                  frame #2 {
                    w523 = -1
                    # "depth"
                    # "altimeter time"
                    # "conductivity"
                    # "temperature"
                    # "time"
                    # "pressure"
                    n196 = Rotate 1D Array(1:w541, 2:w523) -> (0:w540:timestamp[])
                    n197 = Get Date/Time In Seconds() -> (seconds since 1Jan1904=w539:timestamp)
                    n198 = Rotate 1D Array(1:w530, 2:w523) -> (0:w538:dbl[])
                    n199 = Rotate 1D Array(1:w531, 2:w523) -> (0:w537:dbl[])
                    n200 = Rotate 1D Array(1:w532, 2:w523) -> (0:w535:dbl[])
                    n201 = Rotate 1D Array(1:w529, 2:w523) -> (0:w527:dbl[])
                    n202 = Rotate 1D Array(1:w526, 2:w523) -> (0:w525:dbl[])
                    n203 = Replace Array Subset(array=w540, new element=w539, index=w516) -> (w511:timestamp[])
                    n204 = Replace Array Subset(array=w538, new element=w528, index=w516) -> (w522:dbl[])
                    n205 = Replace Array Subset(array=w537, new element=w536, index=w516) -> (w520:dbl[])
                    n206 = Replace Array Subset(array=w535, new element=w534, index=w516) -> (w517:dbl[])
                    n207 = Replace Array Subset(array=w527, new element=w533, index=w516) -> (w515:dbl[])
                    n208 = Replace Array Subset(array=w525, new element=w524, index=w516) -> (w513:dbl[])
                    n209 = Build Cluster Array(w511, w522) -> (→"Pressure":T1)
                    n210 = Build Cluster Array(w511, w520) -> (→"Temperature":T1)
                    n211 = Build Cluster Array(w511, w517) -> (→"Conductivity":T1)
                    n212 = Multiply(x=w513, y=750.0) -> (x*y=w512:dbl[])
                    n213 = Build Cluster Array(w511, w512) -> (→"Alti Range":T1)
                  }
                  frame #3 {
                    n214 = Array Size(array=w545) -> (size(s)=w543:i32)
                    n215 = Greater?(x=w543, y=1) -> (0:w542:bool)
                    n216 = case shown="True" w542 {
                      tunnel: w545 -> [_ w562]
                      tunnel: w543 -> [_ w559]
                      tunnel: w544 -> [_ w555]
                      frame False {
                      }
                      frame True {
                        w556 = 0
                        w557 = 1
                        n217 = Subtract(x=w559, y=w557) -> (x-y=w558:i32)
                        n218 = Array Subset(array=w562, index=w557, length=w558) -> (w561:dbl[])
                        n219 = Array Subset(array=w562, index=w556, length=w558) -> (w560:dbl[])
                        n220 = Subtract(x=w561, y=w560) -> (x-y=w549:dbl[])
                        n221 = Array Subset(array=w555, index=w557, length=w558) -> (w551:timestamp[])
                        n222 = Array Subset(array=w555, index=w556, length=w558) -> (w553:timestamp[])
                        n223 = To Double Precision Float(number=w551) -> (double precision float=w550:dbl[])
                        n224 = To Double Precision Float(number=w553) -> (double precision float=w552:dbl[])
                        n225 = Subtract(x=w550, y=w552) -> (x-y=w554:dbl[])
                        n226 = Divide(x=w549, y=w554) -> (x/y=w547:dbl[])
                        n227 = Build Cluster Array(w551, w547) -> (→"Dz/Dt":T1)
                      }
                    }
                  }
                }
                n228 = case shown="True" w469 {
                  tunnel: w466 -> [_ w565]
                  frame False {
                  }
                  frame True {
                    n229 = Get Date/Time In Seconds() -> (seconds since 1Jan1904=→"Time @ max":timestamp)
                    n230 = property on="Payout" class="Slide (strict)"() -> ("Value"=→"Max payout":dbl)  [unwired: 2 in, 2 out]
                    "Max depth" <- w565
                  }
                }
                n231 = case shown="False" w468 {
                  frame False {
                    n232 = property on="Max depth" class="DigNum (strict)"("Value"=0.0) -> ()  [unwired: 2 in, 2 out]
                  }
                  frame True {
                  }
                }
              }
              frame True {
                # "If CTD is emtpy string: increment CTD Miss count, and blink CTD bar"
                n233 = property on="CTD Com Miss Count" class="DigNum (strict)"() -> ("Value"=w576:dbl)  [unwired: 2 in, 2 out]
                n234 = Increment(x=w576) -> (x+1=w574:dbl)
                n235 = Greater?(x=w574, y=1) -> (0:w566:bool)
                n236 = property on="Depth" class="Slide (strict)"("Blinking"=w566) -> ()  [unwired: 2 in, 2 out]
                n237 = property on="CTD data" class="Str"("Blinking"=w566) -> ()  [unwired: 2 in, 2 out]
                n238 = property on="CTD Com Miss Count" class="DigNum (strict)"("Value"=w574) -> ()  [unwired: 2 in, 2 out]
                n239 = property on="Pressure" class="XYGraph (strict)"("Blinking"=w566) -> ()  [unwired: 2 in, 2 out]
                n240 = property on="Conductivity" class="XYGraph (strict)"("Blinking"=w566) -> ()  [unwired: 2 in, 2 out]
                n241 = property on="Temperature" class="XYGraph (strict)"("Blinking"=w566) -> ()  [unwired: 2 in, 2 out]
                n242 = property on="Dz/Dt" class="XYGraph (strict)"("Blinking"=w566) -> ()  [unwired: 2 in, 2 out]
              }
            }
          }
        }
      }
      frame #7 {
        # "Check for dead com links"
        n243 = stacked-sequence {
          seq-local: [w583 _] -> [_ w600]
          tunnel: w581 -> [w584 _]
          tunnel: [_ w600] -> w580
          tunnel: w579 -> [_ w601]
          tunnel: [_ w599] -> w578
          tunnel: w577 -> [w582 _]
          frame #0 {
            # "If winch miss count > 25, close connection and open again"
            n244 = property on="Winch Com Miss Count" class="DigNum (strict)"() -> ("Value"=w587:dbl)  [unwired: 2 in, 2 out]
            n245 = Greater?(x=w587, y=25) -> (0:w585:bool)
            n246 = case shown="True" w585 {
              tunnel: w584 -> [w588 w591]
              tunnel: [w588 w590] -> w583
              tunnel: w582 -> [_ w589]
              frame False {
              }
              frame True {
                n247 = stacked-sequence {
                  tunnel: w591 -> [w593 _ _]
                  tunnel: [_ _ w596] -> w590
                  tunnel: w589 -> [_ _ w594]
                  frame #0 {
                    n248 = TCP Close Connection(connection ID=w593) -> (error out=w592:errorcluster)  [unwired: 2 in, 1 out]
                    n249 = call <vilib>:"Clear Errors.vi"("error in (no error)"=w592) -> ()  [unwired: 5 in, 2 out]
                  }
                  frame #1 {
                    n250 = call "Time Delay"() -> ()  [unwired: 11 in, 1 out]
                  }
                  frame #2 {
                    n251 = TCP Open Connection(address=w594, remote port or service name=4050, timeout ms (60000)=1000) -> (connection ID=w596:refnum<k5>, error out=w595:errorcluster)  [unwired: 2 in]
                    n252 = call <vilib>:"Clear Errors.vi"("error in (no error)"=w595) -> ()  [unwired: 5 in, 2 out]
                  }
                }
              }
            }
          }
          frame #1 {
            # "If CTD miss count > 10, close connection and open again"
            n253 = property on="CTD Com Miss Count" class="DigNum (strict)"() -> ("Value"=w602:dbl)  [unwired: 2 in, 2 out]
            n254 = Greater?(x=w602, y=10) -> (0:w604:bool)
            n255 = case shown="True" w604 {
              tunnel: w601 -> [w605 w607]
              tunnel: [w605 w606] -> w599
              frame False {
              }
              frame True {
                n256 = stacked-sequence {
                  tunnel: w607 -> [w609 _ _ _]
                  tunnel: [_ _ _ w614] -> w606
                  frame #0 {
                    n257 = TCP Close Connection(connection ID=w609) -> (error out=w608:errorcluster)  [unwired: 2 in, 1 out]
                    n258 = call <vilib>:"Clear Errors.vi"("error in (no error)"=w608) -> ()  [unwired: 5 in, 2 out]
                  }
                  frame #1 {
                    n259 = call "Time Delay2"() -> ()  [unwired: 11 in, 1 out]
                  }
                  frame #2 {
                    n260 = property on="CTD Com Miss Count" class="DigNum (strict)"("Value"=0) -> ()  [unwired: 2 in, 2 out]
                  }
                  frame #3 {
                    n261 = property on="Port" class="DigNum (strict)"() -> ("Value"=w612:i32)  [unwired: 2 in, 2 out]
                    n262 = property on="CTD Data  IP Address" class="Str"() -> ("Value"=w613:string)  [unwired: 2 in, 2 out]
                    n263 = TCP Open Connection(address=w613, remote port or service name=w612, timeout ms (60000)=1000) -> (connection ID=w614:refnum<k5>, error out=w611:errorcluster)  [unwired: 2 in]
                    n264 = call <vilib>:"Clear Errors.vi"("error in (no error)"=w611) -> ()  [unwired: 5 in, 2 out]
                  }
                }
              }
            }
          }
        }
      }
      frame #8 {
        # "Check if the values set by the user \nand the values on the controls are the same"
        # "Image Capture of the Front Panel"
        n265 = property on="Enabled" class="Bool (strict)"() -> ("Value"=w622:bool)  [unwired: 2 in, 2 out]
        n266 = case shown="True" w622 {
          frame False {
          }
          frame True {
            n267 = property on="Min Payout" class="DigNum (strict)"() -> ("Value"=w681:dbl)  [unwired: 2 in, 2 out]
            n268 = property on="Min. payout [turns]" class="DigNum (strict)"() -> ("Value"=w680:dbl)  [unwired: 2 in, 2 out]
            n269 = property on="Wire In Speed" class="DigNum (strict)"() -> ("Value"=w673:dbl)  [unwired: 2 in, 2 out]
            n270 = property on="Wire In Speed\n[turns/sec]" class="DigNum (strict)"() -> ("Value"=w672:dbl)  [unwired: 2 in, 2 out]
            n271 = property on="Max. payout [turns]" class="DigNum (strict)"() -> ("Value"=w679:dbl)  [unwired: 2 in, 2 out]
            n272 = property on="Max Payout" class="DigNum (strict)"() -> ("Value"=w678:dbl)  [unwired: 2 in, 2 out]
            n273 = property on="Wire Out Speed\n[turns/sec]" class="DigNum (strict)"() -> ("Value"=w676:dbl)  [unwired: 2 in, 2 out]
            n274 = property on="Wire Out Speed" class="DigNum (strict)"() -> ("Value"=w675:dbl)  [unwired: 2 in, 2 out]
            n275 = Not Equal?(x=w680, y=w681) -> (x != y?=w682:bool)
            n276 = Not Equal?(x=w673, y=w672) -> (x != y?=w671:bool)
            n277 = Not Equal?(x=w679, y=w678) -> (x != y?=w677:bool)
            n278 = Not Equal?(x=w676, y=w675) -> (x != y?=w674:bool)
            n279 = property on="Min. payout [turns]" class="DigNum (strict)"("Blinking"=w682) -> ()  [unwired: 2 in, 2 out]
            n280 = property on="Min Payout" class="DigNum (strict)"("Blinking"=w682) -> ()  [unwired: 2 in, 2 out]
            n281 = property on="Wire In Speed\n[turns/sec]" class="DigNum (strict)"("Blinking"=w671) -> ()  [unwired: 2 in, 2 out]
            n282 = property on="Max. payout [turns]" class="DigNum (strict)"("Blinking"=w677) -> ()  [unwired: 2 in, 2 out]
            n283 = property on="Wire Out Speed\n[turns/sec]" class="DigNum (strict)"("Blinking"=w674) -> ()  [unwired: 2 in, 2 out]
            n284 = property on="Wire In Speed" class="DigNum (strict)"("Blinking"=w671) -> ()  [unwired: 2 in, 2 out]
            n285 = property on="Max Payout" class="DigNum (strict)"("Blinking"=w677) -> ()  [unwired: 2 in, 2 out]
            n286 = property on="Wire Out Speed" class="DigNum (strict)"("Blinking"=w674) -> ()  [unwired: 2 in, 2 out]
            n287 = property on="Stop decel out" class="DigNum (strict)"() -> ("Value"=w649:dbl)  [unwired: 2 in, 2 out]
            n288 = property on="Decel Stop Out" class="DigNum (strict)"() -> ("Value"=w648:dbl)  [unwired: 2 in, 2 out]
            n289 = property on="Final in Speed" class="DigNum (strict)"() -> ("Value"=w670:dbl)  [unwired: 2 in, 2 out]
            n290 = property on="Final In Speed\n[turns/sec]" class="DigNum (strict)"() -> ("Value"=w669:dbl)  [unwired: 2 in, 2 out]
            n291 = property on="Acc In" class="DigNum (strict)"() -> ("Value"=w664:dbl)  [unwired: 2 in, 2 out]
            n292 = property on="Accel  in" class="DigNum (strict)"() -> ("Value"=w663:dbl)  [unwired: 2 in, 2 out]
            n293 = property on="Acc Out" class="DigNum (strict)"() -> ("Value"=w661:dbl)  [unwired: 2 in, 2 out]
            n294 = property on="Accel out" class="DigNum (strict)"() -> ("Value"=w660:dbl)  [unwired: 2 in, 2 out]
            n295 = Not Equal?(x=w649, y=w648) -> (x != y?=w647:bool)
            n296 = Not Equal?(x=w670, y=w669) -> (x != y?=w668:bool)
            n297 = Not Equal?(x=w664, y=w663) -> (x != y?=w662:bool)
            n298 = Not Equal?(x=w661, y=w660) -> (x != y?=w659:bool)
            n299 = property on="Stop decel out" class="DigNum (strict)"("Blinking"=w647) -> ()  [unwired: 2 in, 2 out]
            n300 = property on="Decel Stop Out" class="DigNum (strict)"("Blinking"=w647) -> ()  [unwired: 2 in, 2 out]
            n301 = property on="Final in Speed" class="DigNum (strict)"("Blinking"=w668) -> ()  [unwired: 2 in, 2 out]
            n302 = property on="Final In Speed\n[turns/sec]" class="DigNum (strict)"("Blinking"=w668) -> ()  [unwired: 2 in, 2 out]
            n303 = property on="Accel  in" class="DigNum (strict)"("Blinking"=w662) -> ()  [unwired: 2 in, 2 out]
            n304 = property on="Accel out" class="DigNum (strict)"("Blinking"=w659) -> ()  [unwired: 2 in, 2 out]
            n305 = property on="Acc In" class="DigNum (strict)"("Blinking"=w662) -> ()  [unwired: 2 in, 2 out]
            n306 = property on="Acc Out" class="DigNum (strict)"("Blinking"=w659) -> ()  [unwired: 2 in, 2 out]
            n307 = property on="Decel Stop In" class="DigNum (strict)"() -> ("Value"=w652:dbl)  [unwired: 2 in, 2 out]
            n308 = property on="Stop decel in" class="DigNum (strict)"() -> ("Value"=w651:dbl)  [unwired: 2 in, 2 out]
            n309 = property on="Decel in" class="DigNum (strict)"() -> ("Value"=w658:dbl)  [unwired: 2 in, 2 out]
            n310 = property on="Decel In" class="DigNum (strict)"() -> ("Value"=w657:dbl)  [unwired: 2 in, 2 out]
            n311 = property on="Decel Out" class="DigNum (strict)"() -> ("Value"=w655:dbl)  [unwired: 2 in, 2 out]
            n312 = property on="Decel out" class="DigNum (strict)"() -> ("Value"=w654:dbl)  [unwired: 2 in, 2 out]
            n313 = property on="Slow Depth" class="DigNum (strict)"() -> ("Value"=w667:dbl)  [unwired: 2 in, 2 out]
            n314 = property on="Slow depth\n[turns]" class="DigNum (strict)"() -> ("Value"=w666:dbl)  [unwired: 2 in, 2 out]
            n315 = Not Equal?(x=w652, y=w651) -> (x != y?=w650:bool)
            n316 = Not Equal?(x=w658, y=w657) -> (x != y?=w656:bool)
            n317 = Not Equal?(x=w655, y=w654) -> (x != y?=w653:bool)
            n318 = Not Equal?(x=w667, y=w666) -> (x != y?=w665:bool)
            n319 = property on="Stop decel in" class="DigNum (strict)"("Blinking"=w650) -> ()  [unwired: 2 in, 2 out]
            n320 = property on="Decel in" class="DigNum (strict)"("Blinking"=w656) -> ()  [unwired: 2 in, 2 out]
            n321 = property on="Decel out" class="DigNum (strict)"("Blinking"=w653) -> ()  [unwired: 2 in, 2 out]
            n322 = property on="Decel Stop In" class="DigNum (strict)"("Blinking"=w650) -> ()  [unwired: 2 in, 2 out]
            n323 = property on="Decel In" class="DigNum (strict)"("Blinking"=w656) -> ()  [unwired: 2 in, 2 out]
            n324 = property on="Decel Out" class="DigNum (strict)"("Blinking"=w653) -> ()  [unwired: 2 in, 2 out]
            n325 = property on="Slow depth\n[turns]" class="DigNum (strict)"("Blinking"=w665) -> ()  [unwired: 2 in, 2 out]
            n326 = property on="Slow Depth" class="DigNum (strict)"("Blinking"=w665) -> ()  [unwired: 2 in, 2 out]
          }
        }
        n327 = Get Date/Time In Seconds() -> (seconds since 1Jan1904=w627:timestamp)
        n328 = Format Date/Time String(seconds (now)=w627) -> (date/time string=w626:string)  [unwired: 2 in]
        n329 = Concatenate Strings("Updated: ", w626) -> (→"Last update string":string)
        n330 = case shown="True" "Screen Capture" {
          frame False {
            n331 = property on="Path of Image Capture" class="Path"("DisabledEnum"=2) -> ()  [unwired: 2 in, 2 out]
          }
          frame True {
            n332 = property on="Path of Image Capture" class="Path"("DisabledEnum"=0) -> ()  [unwired: 2 in, 2 out]
            n333 = feedback #1() -> (w684:errorcluster)  [unwired: 1 in]
            n334 = call <vilib>:"Check if File or Folder Exists.vi"("error in (no error)"=w684, "path"="Path of Image Capture") -> ("error out"=w686:errorcluster, "file or folder exists?"=w688:bool, "dup path"=w689:path)  [unwired: 7 in]
            n335 = case shown="True" w688 {
              tunnel: w689 -> [w697 w699]
              tunnel: w686 -> [w692 _]
              tunnel: [w691 w698] -> w685
              frame False {
                n336 = Open/Create/Replace File(file path (use dialog)=w697, error in=w692, operation (0:open)=4, access (0:read/write)=0) -> (refnum out=w693:refnum<file>, error out=w694:errorcluster)  [unwired: 2 in, 1 out]
                n337 = Close File(refnum=w693, error in=w694) -> (error out=w691:errorcluster)  [unwired: 1 out]
              }
              frame True {
                # "Close VI ref"
                # "24 bit image depth"
                # "Open VI Reference Function"
                # "Current VI's Path"
                # "Save an image capture of the Fron Panel"
                n338 = Current VI's Path() -> (path=w706:path)
                n339 = Open VI Reference(vi path=w706) -> (vi reference=w703:refnum<vi>, error out=w705:errorcluster)  [unwired: 5 in]
                n340 = invoke class="VI" method="FP.Get Image"(reference=w703, error in=w705, "image depth"=24) -> (reference out=w701:refnum<vi>, error out=w702:errorcluster, "image data"=w704:T6)  [unwired: 3 in, 3 out]
                n341 = Close Reference(reference=w701) -> ()  [unwired: 1 in, 1 out]
                n342 = call <vilib>:"Write PNG File.vi"("error in (no error)"=w702, "image data"=w704, "path to PNG file"=w699) -> ("error out"=w698:errorcluster)  [unwired: 7 in, 1 out]
              }
            }
            n343 = feedback-in #1(w685) -> ()
          }
        }
        n344 = To Double Precision Float(number=w621) -> (double precision float=w618:dbl[])
        n345 = To Double Precision Float(number=w620) -> (double precision float=w619:dbl[])
        n346 = stacked-sequence {
          tunnel: w619 -> [_ w634 w643]
          tunnel: w618 -> [_ w635 w645]
          tunnel: w617 -> [w631 w636 _]
          tunnel: w616 -> [w630 w633 _]
          frame #0 {
            n347 = Build Array(w631, w630) -> (w632:dbl[][])
            n348 = Array Max & Min(array=w632) -> (max value=w629:dbl, min value=w628:dbl)  [unwired: 2 out]
            n349 = property on="Depth History" class="XYGraph (strict)"("YScale.Minimum"=w628) -> ()  [unwired: 2 in, 2 out]
            n350 = property on="Depth History" class="XYGraph (strict)"("YScale.Maximum"=w629) -> ()  [unwired: 2 in, 2 out]
          }
          frame #1 {
            n351 = Build Cluster Array(w635, w636) -> (w638:cluster{"seconds since 1Jan1904":dbl, dbl}[])
            n352 = Bundle(w638) -> (w640:T7)  [unwired: 1 in]
            n353 = Build Cluster Array(w634, w633) -> (w637:cluster{"seconds since 1Jan1904":dbl, dbl}[])
            n354 = Bundle(w637) -> (w641:T7)  [unwired: 1 in]
            n355 = Build Array(w640, w641) -> (→"Depth History":T2)
          }
          frame #2 {
            n356 = Build Array(w645, w643) -> (w646:dbl[][])
            n357 = Array Max & Min(array=w646) -> (max value=w642:dbl, min value=w644:dbl)  [unwired: 2 out]
            n358 = property on="Dz/Dt" class="XYGraph (strict)"("XScale.Minimum"=w644) -> ()  [unwired: 2 in, 2 out]
            n359 = property on="Pressure" class="XYGraph (strict)"("XScale.Minimum"=w644) -> ()  [unwired: 2 in, 2 out]
            n360 = property on="Conductivity" class="XYGraph (strict)"("XScale.Minimum"=w644) -> ()  [unwired: 2 in, 2 out]
            n361 = property on="Alti Range" class="XYGraph (strict)"("XScale.Minimum"=w644) -> ()  [unwired: 2 in, 2 out]
            n362 = property on="Temperature" class="XYGraph (strict)"("XScale.Minimum"=w644) -> ()  [unwired: 2 in, 2 out]
            n363 = property on="Depth History" class="XYGraph (strict)"("XScale.Minimum"=w644) -> ()  [unwired: 2 in, 2 out]
            n364 = property on="Pressure" class="XYGraph (strict)"("XScale.Maximum"=w642) -> ()  [unwired: 2 in, 2 out]
            n365 = property on="Depth History" class="XYGraph (strict)"("XScale.Maximum"=w642) -> ()  [unwired: 2 in, 2 out]
            n366 = property on="Temperature" class="XYGraph (strict)"("XScale.Maximum"=w642) -> ()  [unwired: 2 in, 2 out]
            n367 = property on="Alti Range" class="XYGraph (strict)"("XScale.Maximum"=w642) -> ()  [unwired: 2 in, 2 out]
            n368 = property on="Conductivity" class="XYGraph (strict)"("XScale.Maximum"=w642) -> ()  [unwired: 2 in, 2 out]
            n369 = property on="Dz/Dt" class="XYGraph (strict)"("XScale.Maximum"=w642) -> ()  [unwired: 2 in, 2 out]
          }
        }
      }
    }
  }
  n370 = Strip Path(path=w15) -> (stripped path=w14:path)  [unwired: 1 out]
  n371 = Strip Path(path=w14) -> (stripped path=w13:path)  [unwired: 1 out]
  n372 = Build Path(base path=w13, name or relative path="Sites") -> (appended path=w11:path)
  n373 = Build Path(base path=w11, name or relative path="FCTD_WINCH") -> (appended path=w9:path)
  n374 = Build Path(base path=w9, name or relative path="LabView.png") -> (appended path=w7:path)
  n375 = property on="Path of Image Capture" class="Path"("Value"=w7) -> ()  [unwired: 2 in, 2 out]
  n376 = TCP Close Connection(connection ID=w24, error in (no error)=w57) -> (error out=w26:errorcluster)  [unwired: 1 in, 1 out]
  n377 = TCP Close Connection(connection ID=w33, error in (no error)=w31) -> (error out=w35:errorcluster)  [unwired: 1 in, 1 out]
  n378 = call <vilib>:"Simple Error Handler.vi"("error in (no error)"=w26) -> ()  [unwired: 4 in, 5 out]
  n379 = call <vilib>:"Simple Error Handler.vi"("error in (no error)"=w35) -> ()  [unwired: 4 in, 5 out]
  "CTD Com Miss Count" <- w25
  "Winch Com Miss Count" <- w25
  "isMaxPaySet" <- FALSE
  "RL Status Received" <- FALSE
